vi "Autonomous Independent.vi"   [LabVIEW 2017]
doc: "This VI is called when autonomous begins, and will automatically be terminated when autonomous ends. You can carry out timed or sensor driven robot movement independently without needing to return to the caller."
uses:
  <vilib>/Rock Robotics/WPI/Utilities/WPI_GetSetVariantRefNum.vi
  <vilib>/Rock Robotics/Network Tables/NT Write Numeric Array.vi
  <vilib>/Rock Robotics/Network Tables/NT Read String.vi
  <vilib>/Rock Robotics/WPI/RobotDrive/WPI_RobotDriveMecanumDrive_Cartesian.vi
panel:
  # "Be sure to right-click and choose Data Operations>>Make Current Value default if you want to save the array values with the VI"
types:
  T1 = typedef "WPI_JoystickDevRef.ctl" = cluster{"Device":T2}
  T2 = typedef "WPI_JoystickDeviceEnum.ctl" = enum16{"USB 0", "USB 1", "USB 2", "USB 3", "USB 4", "USB 5"}
  T3 = typedef "WPI_RobotDriveDevRef.ctl" = cluster{"DevStatus":errorcluster, "Motors[]":T4[], "Square Inputs":bool, "Max Output":dbl}
  T4 = typedef "WPI_MotorControlDeviceRef.ctl" = cluster{"DeviceStatus":errorcluster, "Type":T5, "PWM":cluster{"PWM Channel":T6, "DeadBand":T7}, "CAN":cluster{"Device Number":u8, "SetOutput VI Ref":variant, "GetOutput VI Ref":variant, "Enable VI Ref":variant, "Disable VI Ref":variant, "Data":variant}, "Invert":bool, "DIO PWM":cluster{"PWM \"Enable\" Channel":T6, "DIOChannel":T8, "PWM Rate":dbl}}
  T5 = typedef "WPI_MotorControlType.ctl" = enum16{"PWM", "CAN", "DIO PWM"}
  T6 = typedef "FPGA_DIOPWMChannel.ctl" = enum8{"PWM 0", "PWM 1", "PWM 2", "PWM 3", "PWM 4", "PWM 5", "PWM 6", "PWM 7", "PWM 8", "PWM 9", "PWM MXP 0", "PWM MXP 1", "PWM MXP 2", "PWM MXP 3", "PWM MXP 4", "PWM MXP 5", "PWM MXP 6", "PWM MXP 7", "PWM MXP 8", "PWM MXP 9", "Invalid"}
  T7 = typedef "WPI_PWMDeadband.ctl" = cluster{"Name":string, "maxPositivePwm":i32, "minPositivePwm":i32, "centerPwm":i32, "maxNegativePwm":i32, "minNegativePwm":i32, "angularRange":u16}
  T8 = typedef "FPGA_DIOChannel.ctl" = enum8{"DIO 0", "DIO 1", "DIO 2", "DIO 3", "DIO 4", "DIO 5", "DIO 6", "DIO 7", "DIO 8", "DIO 9", "DIO MXP 0", "DIO MXP 1", "DIO MXP 2", "DIO MXP 3", "DIO MXP 4", "DIO MXP 5", "DIO MXP 6", "DIO MXP 7", "DIO MXP 8", "DIO MXP 9", "DIO MXP 10", "DIO MXP 11", "DIO MXP 12", "DIO MXP 13", "DIO MXP 14", "DIO MXP 15", "SPI Port CS1", "SPI Port CS2", "SPI Port CS3", "SPI Port MISO", "SPI Port MOSI", "Invalid"}
  T9 = cluster{"RobotDriveDevRef":T3, "error out":errorcluster}
  T10 = cluster{"RobotDriveDevRef 2":T3, "error out":errorcluster}
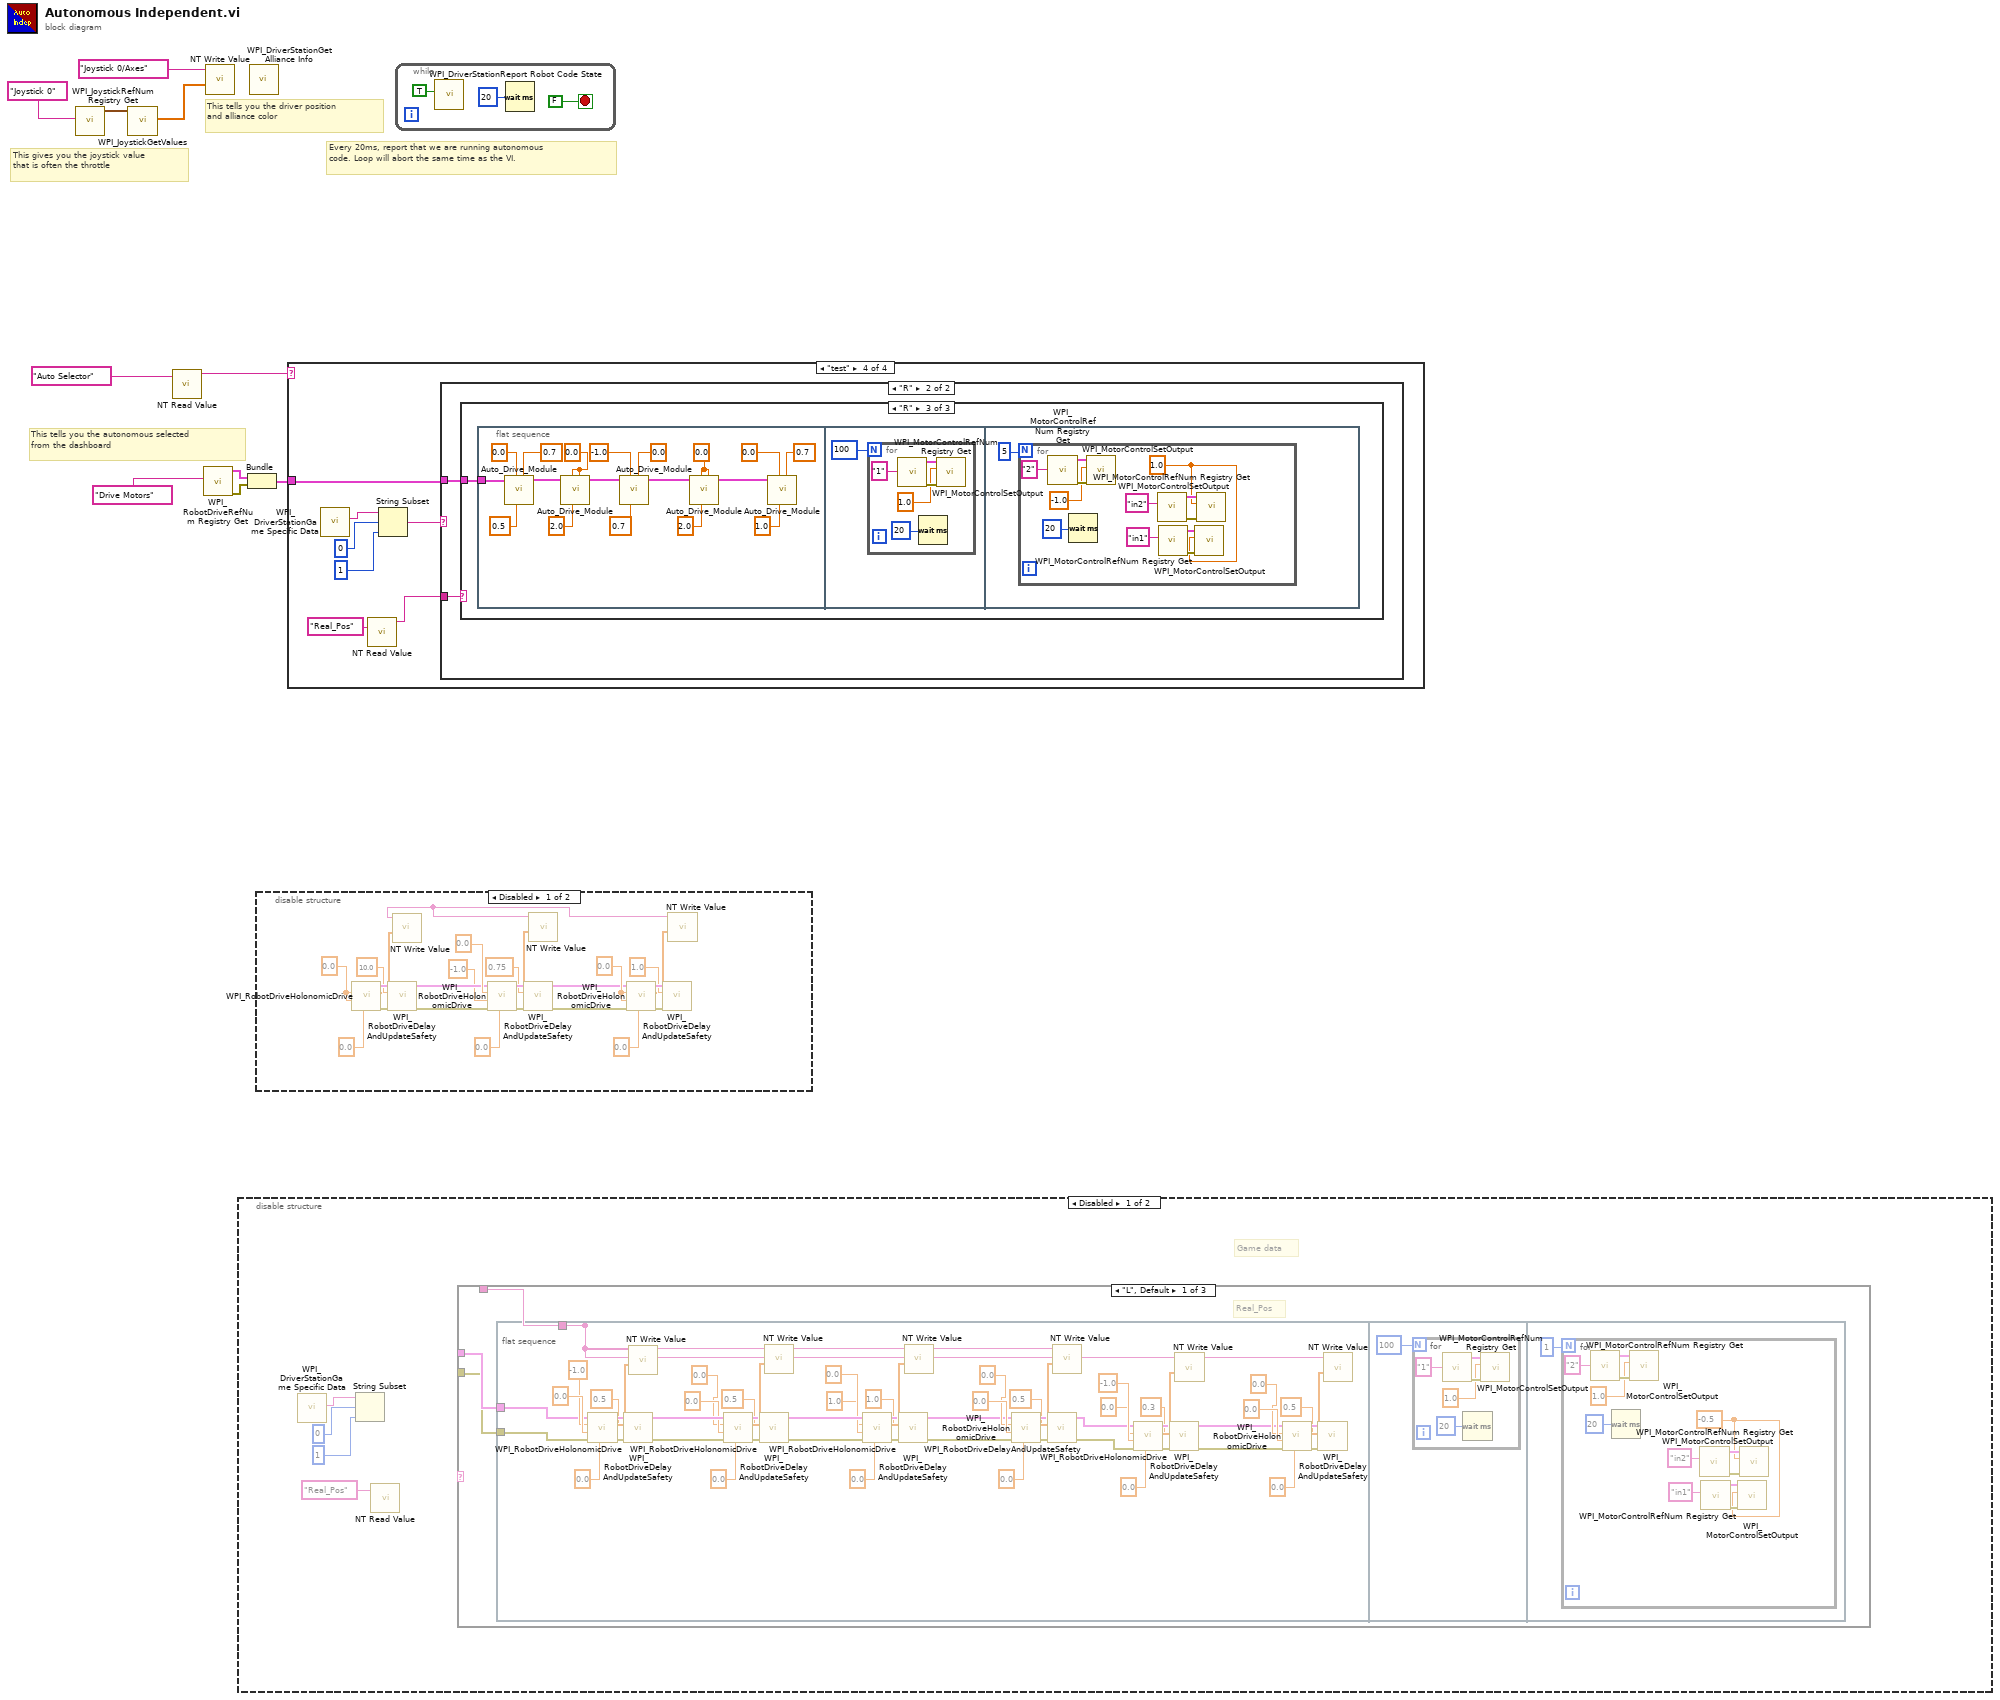
[diagram p0: block diagram]
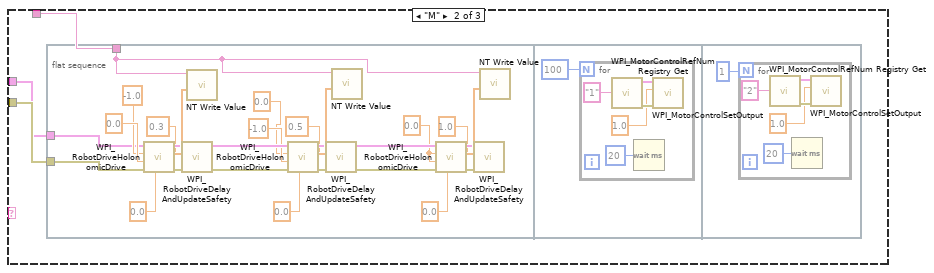
[diagram p2: hidden frame]
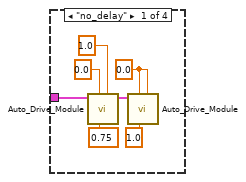
[diagram p6: hidden frame]
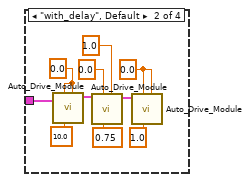
[diagram p7: hidden frame]
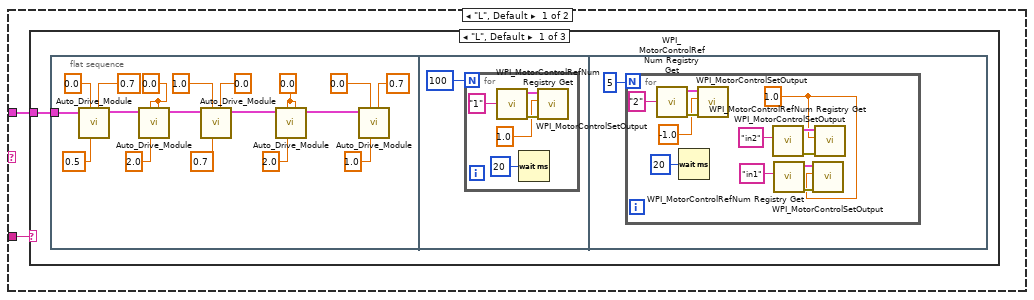
[diagram p9: hidden frame]
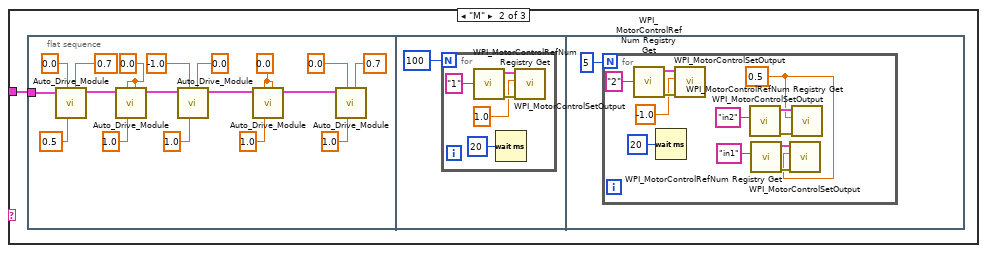
[diagram p10: hidden frame]
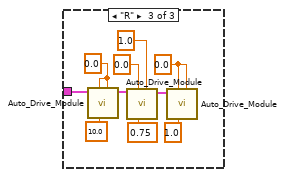
[diagram p11: hidden frame]
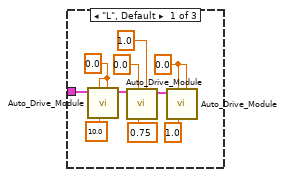
[diagram p12: hidden frame]
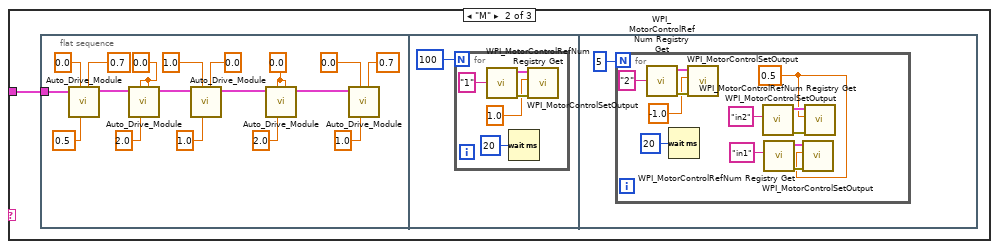
[diagram p13: hidden frame]
diagram:
  # "This tells you the autonomous selected\nfrom the dashboard"
  # "Every 20ms, report that we are running autonomous\ncode. Loop will abort the same time as the VI."
  # "This tells you the driver position\nand alliance color"
  # "This gives you the joystick value\nthat is often the throttle"
  n1 = call <vilib>:"WPI_JoystickRefNum Registry Get.vi"("refnum name"="Joystick 0") -> ("JoystickDevRef"=w8:T1)  [unwired: 1 in, 9 out]
  n2 = call <vilib>:"WPI_JoystickGetValues.vi"("JoystickDevRef"=w8) -> ("Axes"=w7:dbl[])  [unwired: 6 in, 4 out]
  n3 = call-poly <vilib>:"NT Read Value.vi"("Name"="Auto Selector") -> ("String"=w4:string)  [unwired: 9 in, 1 out]
  n4 = call <vilib>:"WPI_RobotDriveRefNum Registry Get.vi"("refnum name"="Drive Motors") -> ("error out"=w3:errorcluster, "RobotDriveDevRef"=w2:T3)  [unwired: 1 in, 8 out]
  n5 = call-poly <vilib>:"NT Write Value.vi"("Numeric Array"=w7, "Name"="Joystick 0/Axes") -> ()  [unwired: 9 in, 1 out]
  n6 = disable-structure shown="Disabled" {
    frame Disabled {
      # "Game data"
      n7 = call <vilib>:"WPI_DriverStationGame Specific Data.vi"() -> ("Game Specific Data"=w12:string)  [unwired: 11 in]
      n8 = String Subset(string=w12, offset (0)=0, length (rest)=1) -> ()  [unwired: 1 out]
      n9 = call-poly <vilib>:"NT Read Value.vi"("Name"="Real_Pos") -> ()  [unwired: 9 in, 2 out]
      n10 = case shown="\"L\", Default" {
        selector: _ -> [_ _ _]
        tunnel: _ -> [w15 w94 _]
        tunnel: _ -> [w16 w93 _]
        tunnel: _ -> [w17 w92 _]
        frame "L", Default {
          # "Real_Pos"
          n11 = flat-sequence {
            tunnel: w15 -> [w51]
            tunnel: w16 -> [w48]
            tunnel: [w19] -> _
            tunnel: w17 -> [w19]
            frame #0 {
              n12 = call-poly <vilib>:"WPI_RobotDriveHolonomicDrive.vi"("Rotation"=0.0, "error in (no error)"=w51, "Y"=0.0, "X"=-1.0, "RobotDriveDevRef"=w48) -> ("error out"=w60:errorcluster, "Motor Values"=w70:dbl[], "RobotDriveDevRef"=w61:T3)  [unwired: 4 in]
              n13 = call <vilib>:"WPI_RobotDriveDelayAndUpdateSafety.vi"("error in (no error)"=w60, "Delay (s)"=0.5, "RobotDriveDevRef"=w61) -> ("error out"=w65:errorcluster, "RobotDriveDevRef 2"=w64:T3)  [unwired: 7 in]
              n14 = call-poly <vilib>:"NT Write Value.vi"("Numeric Array"=w70, "Name"=w19) -> ()  [unwired: 9 in, 1 out]
              n15 = call-poly <vilib>:"WPI_RobotDriveHolonomicDrive.vi"("Rotation"=0.0, "error in (no error)"=w65, "Y"=0.0, "X"=0.0, "RobotDriveDevRef"=w64) -> ("error out"=w62:errorcluster, "Motor Values"=w71:dbl[], "RobotDriveDevRef"=w63:T3)  [unwired: 4 in]
              n16 = call <vilib>:"WPI_RobotDriveDelayAndUpdateSafety.vi"("error in (no error)"=w62, "Delay (s)"=0.5, "RobotDriveDevRef"=w63) -> ("error out"=w69:errorcluster, "RobotDriveDevRef 2"=w68:T3)  [unwired: 7 in]
              n17 = call-poly <vilib>:"NT Write Value.vi"("Numeric Array"=w71, "Name"=w19) -> ()  [unwired: 9 in, 1 out]
              n18 = call-poly <vilib>:"WPI_RobotDriveHolonomicDrive.vi"("Rotation"=0.0, "error in (no error)"=w69, "Y"=0.0, "X"=1.0, "RobotDriveDevRef"=w68) -> ("error out"=w66:errorcluster, "Motor Values"=w72:dbl[], "RobotDriveDevRef"=w67:T3)  [unwired: 4 in]
              n19 = call <vilib>:"WPI_RobotDriveDelayAndUpdateSafety.vi"("error in (no error)"=w66, "Delay (s)"=1.0, "RobotDriveDevRef"=w67) -> ("error out"=w39:errorcluster, "RobotDriveDevRef 2"=w40:T3)  [unwired: 7 in]
              n20 = call-poly <vilib>:"NT Write Value.vi"("Numeric Array"=w72, "Name"=w19) -> ()  [unwired: 9 in, 1 out]
              n21 = call-poly <vilib>:"WPI_RobotDriveHolonomicDrive.vi"("Rotation"=0.0, "error in (no error)"=w39, "Y"=0.0, "X"=0.0, "RobotDriveDevRef"=w40) -> ("error out"=w45:errorcluster, "Motor Values"=w47:dbl[], "RobotDriveDevRef"=w46:T3)  [unwired: 4 in]
              n22 = call <vilib>:"WPI_RobotDriveDelayAndUpdateSafety.vi"("error in (no error)"=w45, "Delay (s)"=0.5, "RobotDriveDevRef"=w46) -> ("error out"=w20:errorcluster, "RobotDriveDevRef 2"=w21:T3)  [unwired: 7 in]
              n23 = call-poly <vilib>:"NT Write Value.vi"("Numeric Array"=w47, "Name"=w19) -> ()  [unwired: 9 in, 1 out]
              n24 = call-poly <vilib>:"WPI_RobotDriveHolonomicDrive.vi"("Rotation"=0.0, "error in (no error)"=w20, "Y"=-1.0, "X"=0.0, "RobotDriveDevRef"=w21) -> ("error out"=w34:errorcluster, "Motor Values"=w36:dbl[], "RobotDriveDevRef"=w35:T3)  [unwired: 4 in]
              n25 = call <vilib>:"WPI_RobotDriveDelayAndUpdateSafety.vi"("error in (no error)"=w34, "Delay (s)"=0.3, "RobotDriveDevRef"=w35) -> ("error out"=w23:errorcluster, "RobotDriveDevRef 2"=w24:T3)  [unwired: 7 in]
              n26 = call-poly <vilib>:"NT Write Value.vi"("Numeric Array"=w36, "Name"=w19) -> ()  [unwired: 9 in, 1 out]
              n27 = call-poly <vilib>:"WPI_RobotDriveHolonomicDrive.vi"("Rotation"=0.0, "error in (no error)"=w23, "Y"=0.0, "X"=0.0, "RobotDriveDevRef"=w24) -> ("error out"=w29:errorcluster, "Motor Values"=w31:dbl[], "RobotDriveDevRef"=w30:T3)  [unwired: 4 in]
              n28 = call <vilib>:"WPI_RobotDriveDelayAndUpdateSafety.vi"("error in (no error)"=w29, "Delay (s)"=0.5, "RobotDriveDevRef"=w30) -> ()  [unwired: 7 in, 2 out]
              n29 = call-poly <vilib>:"NT Write Value.vi"("Numeric Array"=w31, "Name"=w19) -> ()  [unwired: 9 in, 1 out]
            }
            frame #1 {
              n30 = for {
                N: 100 -> [_]
                n31 = call <vilib>:"WPI_MotorControlRefNum Registry Get.vi"("refnum name"="1") -> ("error out"=w76:errorcluster, "MotorControlDevRef"=w75:T4)  [unwired: 9 in]
                n32 = Wait (ms)(milliseconds to wait=u32 20) -> ()  [unwired: 1 out]
                n33 = call <vilib>:"WPI_MotorControlSetOutput.vi"("error in (no error)"=w76, "Output"=1.0, "MotorControlDevRef"=w75) -> ()  [unwired: 6 in, 3 out]
              }
            }
            frame #2 {
              n34 = for {
                N: 1 -> [_]
                w82 = -0.5
                n35 = call <vilib>:"WPI_MotorControlRefNum Registry Get.vi"("refnum name"="2") -> ("error out"=w89:errorcluster, "MotorControlDevRef"=w87:T4)  [unwired: 9 in]
                n36 = Wait (ms)(milliseconds to wait=u32 20) -> ()  [unwired: 1 out]
                n37 = call <vilib>:"WPI_MotorControlSetOutput.vi"("error in (no error)"=w89, "Output"=1.0, "MotorControlDevRef"=w87) -> ()  [unwired: 6 in, 3 out]
                n38 = call <vilib>:"WPI_MotorControlRefNum Registry Get.vi"("refnum name"="in2") -> ("error out"=w84:errorcluster, "MotorControlDevRef"=w83:T4)  [unwired: 9 in]
                n39 = call <vilib>:"WPI_MotorControlRefNum Registry Get.vi"("refnum name"="in1") -> ("error out"=w86:errorcluster, "MotorControlDevRef"=w85:T4)  [unwired: 9 in]
                n40 = call <vilib>:"WPI_MotorControlSetOutput.vi"("error in (no error)"=w86, "Output"=w82, "MotorControlDevRef"=w85) -> ()  [unwired: 6 in, 3 out]
                n41 = call <vilib>:"WPI_MotorControlSetOutput.vi"("error in (no error)"=w84, "Output"=w82, "MotorControlDevRef"=w83) -> ()  [unwired: 6 in, 3 out]
              }
            }
          }
        }
        frame "M" {
          n42 = flat-sequence {
            tunnel: w94 -> [w99]
            tunnel: w93 -> [w96]
            tunnel: w92 -> [w95]
            frame #0 {
              w106 = 0.0
              n43 = call-poly <vilib>:"WPI_RobotDriveHolonomicDrive.vi"("Rotation"=0.0, "error in (no error)"=w99, "Y"=0.0, "X"=-1.0, "RobotDriveDevRef"=w96) -> ("error out"=w109:errorcluster, "Motor Values"=w119:dbl[], "RobotDriveDevRef"=w110:T3)  [unwired: 4 in]
              n44 = call <vilib>:"WPI_RobotDriveDelayAndUpdateSafety.vi"("error in (no error)"=w109, "Delay (s)"=0.3, "RobotDriveDevRef"=w110) -> ("error out"=w114:errorcluster, "RobotDriveDevRef 2"=w113:T3)  [unwired: 7 in]
              n45 = call-poly <vilib>:"NT Write Value.vi"("Numeric Array"=w119, "Name"=w95) -> ()  [unwired: 9 in, 1 out]
              n46 = call-poly <vilib>:"WPI_RobotDriveHolonomicDrive.vi"("Rotation"=0.0, "error in (no error)"=w114, "Y"=-1.0, "X"=0.0, "RobotDriveDevRef"=w113) -> ("error out"=w111:errorcluster, "Motor Values"=w120:dbl[], "RobotDriveDevRef"=w112:T3)  [unwired: 4 in]
              n47 = call <vilib>:"WPI_RobotDriveDelayAndUpdateSafety.vi"("error in (no error)"=w111, "Delay (s)"=0.5, "RobotDriveDevRef"=w112) -> ("error out"=w118:errorcluster, "RobotDriveDevRef 2"=w117:T3)  [unwired: 7 in]
              n48 = call-poly <vilib>:"NT Write Value.vi"("Numeric Array"=w120, "Name"=w95) -> ()  [unwired: 9 in, 1 out]
              n49 = call-poly <vilib>:"WPI_RobotDriveHolonomicDrive.vi"("Rotation"=0.0, "error in (no error)"=w118, "Y"=w106, "X"=w106, "RobotDriveDevRef"=w117) -> ("error out"=w115:errorcluster, "Motor Values"=w121:dbl[], "RobotDriveDevRef"=w116:T3)  [unwired: 4 in]
              n50 = call <vilib>:"WPI_RobotDriveDelayAndUpdateSafety.vi"("error in (no error)"=w115, "Delay (s)"=1.0, "RobotDriveDevRef"=w116) -> ()  [unwired: 7 in, 2 out]
              n51 = call-poly <vilib>:"NT Write Value.vi"("Numeric Array"=w121, "Name"=w95) -> ()  [unwired: 9 in, 1 out]
            }
            frame #1 {
              n52 = for {
                N: 100 -> [_]
                n53 = call <vilib>:"WPI_MotorControlRefNum Registry Get.vi"("refnum name"="1") -> ("error out"=w125:errorcluster, "MotorControlDevRef"=w124:T4)  [unwired: 9 in]
                n54 = Wait (ms)(milliseconds to wait=u32 20) -> ()  [unwired: 1 out]
                n55 = call <vilib>:"WPI_MotorControlSetOutput.vi"("error in (no error)"=w125, "Output"=1.0, "MotorControlDevRef"=w124) -> ()  [unwired: 6 in, 3 out]
              }
            }
            frame #2 {
              n56 = for {
                N: 1 -> [_]
                n57 = call <vilib>:"WPI_MotorControlRefNum Registry Get.vi"("refnum name"="2") -> ("error out"=w131:errorcluster, "MotorControlDevRef"=w129:T4)  [unwired: 9 in]
                n58 = Wait (ms)(milliseconds to wait=u32 20) -> ()  [unwired: 1 out]
                n59 = call <vilib>:"WPI_MotorControlSetOutput.vi"("error in (no error)"=w131, "Output"=1.0, "MotorControlDevRef"=w129) -> ()  [unwired: 6 in, 3 out]
              }
            }
          }
        }
        frame "R" {
        }
      }
    }
    frame Enabled {
    }
  }
  n60 = Bundle("RobotDriveDevRef"=w2, "error out"=w3) -> (w1:T9)  [unwired: 1 in]
  n61 = call <vilib>:"WPI_DriverStationGet Alliance Info.vi"() -> ()  [unwired: 12 out]
  n62 = disable-structure shown="Disabled" {
    frame Disabled {
      w140 = 0.0
      w153 = 0.0
      n63 = call-poly <vilib>:"WPI_RobotDriveHolonomicDrive.vi"("Rotation"=0.0, "Y"=w153, "X"=w153) -> ("error out"=w159:errorcluster, "Motor Values"=w137:dbl[], 3:"RobotDriveDevRef"=w158:T3, "error in (no error)"=w155:errorcluster, 11:"RobotDriveDevRef"=w154:T3)  [unwired: 4 in]
      n64 = call <vilib>:"WPI_RobotDriveDelayAndUpdateSafety.vi"("error in (no error)"=w159, "Delay (s)"=10.0, "RobotDriveDevRef"=w158) -> ("error out"=w146:errorcluster, "RobotDriveDevRef 2"=w147:T3)  [unwired: 7 in]
      n65 = call-poly <vilib>:"NT Write Value.vi"("Numeric Array"=w137) -> ("Name"=w134:string)  [unwired: 9 in, 1 out]
      n66 = call-poly <vilib>:"WPI_RobotDriveHolonomicDrive.vi"("Rotation"=0.0, "error in (no error)"=w146, "Y"=-1.0, "X"=0.0, "RobotDriveDevRef"=w147) -> ("error out"=w152:errorcluster, "Motor Values"=w136:dbl[], "RobotDriveDevRef"=w151:T3)  [unwired: 4 in]
      n67 = call <vilib>:"WPI_RobotDriveDelayAndUpdateSafety.vi"("error in (no error)"=w152, "Delay (s)"=0.75, "RobotDriveDevRef"=w151) -> ("error out"=w138:errorcluster, "RobotDriveDevRef 2"=w139:T3)  [unwired: 7 in]
      n68 = call-poly <vilib>:"NT Write Value.vi"("Numeric Array"=w136, "Name"=w134) -> ()  [unwired: 9 in, 1 out]
      n69 = call-poly <vilib>:"WPI_RobotDriveHolonomicDrive.vi"("Rotation"=0.0, "error in (no error)"=w138, "Y"=w140, "X"=w140, "RobotDriveDevRef"=w139) -> ("error out"=w144:errorcluster, "Motor Values"=w135:dbl[], "RobotDriveDevRef"=w143:T3)  [unwired: 4 in]
      n70 = call <vilib>:"WPI_RobotDriveDelayAndUpdateSafety.vi"("error in (no error)"=w144, "Delay (s)"=1.0, "RobotDriveDevRef"=w143) -> ()  [unwired: 7 in, 2 out]
      n71 = call-poly <vilib>:"NT Write Value.vi"("Numeric Array"=w135, "Name"=w134) -> ()  [unwired: 9 in, 1 out]
    }
    frame Enabled {
    }
  }
  n72 = case shown="\"test\"" w4 {
    tunnel: w1 -> [w160 w167 _ w177]
    frame "no_delay" {
      w161 = 0.0
      n73 = call "Auto_Drive_Module.vi"("Y"=1.0, "Lasting Time"=0.75, "X"=0.0, "DevRef & Err in"=w160) -> ("DevRef & Err out"=w166:T10)  [unwired: 7 in]
      n74 = call "Auto_Drive_Module.vi"("Y"=w161, "Lasting Time"=1.0, "X"=w161, "DevRef & Err in"=w166) -> ()  [unwired: 7 in, 1 out]
    }
    frame "with_delay", Default {
      w168 = 0.0
      w171 = 0.0
      n75 = call "Auto_Drive_Module.vi"("Y"=w171, "Lasting Time"=10.0, "X"=w171, "DevRef & Err in"=w167) -> ("DevRef & Err out"=w176:T10)  [unwired: 7 in]
      n76 = call "Auto_Drive_Module.vi"("Y"=1.0, "Lasting Time"=0.75, "X"=0.0, "DevRef & Err in"=w176) -> ("DevRef & Err out"=w175:T10)  [unwired: 7 in]
      n77 = call "Auto_Drive_Module.vi"("Y"=w168, "Lasting Time"=1.0, "X"=w168, "DevRef & Err in"=w175) -> ()  [unwired: 7 in, 1 out]
    }
    frame "stay" {
    }
    frame "test" {
      n78 = call <vilib>:"WPI_DriverStationGame Specific Data.vi"() -> ("Game Specific Data"=w181:string)  [unwired: 11 in]
      n79 = call-poly <vilib>:"NT Read Value.vi"("Name"="Real_Pos") -> ("String"=w178:string)  [unwired: 9 in, 1 out]
      n80 = String Subset(string=w181, offset (0)=0, length (rest)=1) -> (substring=w179:string)
      n81 = case shown="\"R\"" w179 {
        tunnel: w178 -> [w185 w273]
        tunnel: w177 -> [w184 w272]
        frame "L", Default {
          n82 = case shown="\"L\", Default" w185 {
            tunnel: w184 -> [w186 w224 w262]
            frame "L", Default {
              n83 = flat-sequence {
                tunnel: w186 -> [w204]
                frame #0 {
                  w189 = 0.0
                  w192 = 0.0
                  n84 = call "Auto_Drive_Module.vi"("Y"=0.7, "Lasting Time"=0.5, "X"=0.0, "DevRef & Err in"=w204) -> ("DevRef & Err out"=w194:T10)  [unwired: 7 in]
                  n85 = call "Auto_Drive_Module.vi"("Y"=w192, "Lasting Time"=2.0, "X"=w192, "DevRef & Err in"=w194) -> ("DevRef & Err out"=w193:T10)  [unwired: 7 in]
                  n86 = call "Auto_Drive_Module.vi"("Y"=0.0, "Lasting Time"=0.7, "X"=1.0, "DevRef & Err in"=w193) -> ("DevRef & Err out"=w187:T10)  [unwired: 7 in]
                  n87 = call "Auto_Drive_Module.vi"("Y"=w189, "Lasting Time"=2.0, "X"=w189, "DevRef & Err in"=w187) -> ("DevRef & Err out"=w188:T10)  [unwired: 7 in]
                  n88 = call "Auto_Drive_Module.vi"("Y"=0.7, "Lasting Time"=1.0, "X"=0.0, "DevRef & Err in"=w188) -> ()  [unwired: 7 in, 1 out]
                }
                frame #1 {
                  n89 = for {
                    N: 100 -> [_]
                    n90 = call <vilib>:"WPI_MotorControlRefNum Registry Get.vi"("refnum name"="1") -> ("error out"=w208:errorcluster, "MotorControlDevRef"=w207:T4)  [unwired: 9 in]
                    n91 = Wait (ms)(milliseconds to wait=u32 20) -> ()  [unwired: 1 out]
                    n92 = call <vilib>:"WPI_MotorControlSetOutput.vi"("error in (no error)"=w208, "Output"=1.0, "MotorControlDevRef"=w207) -> ()  [unwired: 6 in, 3 out]
                  }
                }
                frame #2 {
                  n93 = for {
                    N: 5 -> [_]
                    w214 = 1.0
                    n94 = call <vilib>:"WPI_MotorControlRefNum Registry Get.vi"("refnum name"="2") -> ("error out"=w221:errorcluster, "MotorControlDevRef"=w219:T4)  [unwired: 9 in]
                    n95 = Wait (ms)(milliseconds to wait=u32 20) -> ()  [unwired: 1 out]
                    n96 = call <vilib>:"WPI_MotorControlSetOutput.vi"("error in (no error)"=w221, "Output"=-1.0, "MotorControlDevRef"=w219) -> ()  [unwired: 6 in, 3 out]
                    n97 = call <vilib>:"WPI_MotorControlRefNum Registry Get.vi"("refnum name"="in2") -> ("error out"=w216:errorcluster, "MotorControlDevRef"=w215:T4)  [unwired: 9 in]
                    n98 = call <vilib>:"WPI_MotorControlRefNum Registry Get.vi"("refnum name"="in1") -> ("error out"=w218:errorcluster, "MotorControlDevRef"=w217:T4)  [unwired: 9 in]
                    n99 = call <vilib>:"WPI_MotorControlSetOutput.vi"("error in (no error)"=w218, "Output"=w214, "MotorControlDevRef"=w217) -> ()  [unwired: 6 in, 3 out]
                    n100 = call <vilib>:"WPI_MotorControlSetOutput.vi"("error in (no error)"=w216, "Output"=w214, "MotorControlDevRef"=w215) -> ()  [unwired: 6 in, 3 out]
                  }
                }
              }
            }
            frame "M" {
              n101 = flat-sequence {
                tunnel: w224 -> [w242]
                frame #0 {
                  w227 = 0.0
                  w230 = 0.0
                  n102 = call "Auto_Drive_Module.vi"("Y"=0.7, "Lasting Time"=0.5, "X"=0.0, "DevRef & Err in"=w242) -> ("DevRef & Err out"=w232:T10)  [unwired: 7 in]
                  n103 = call "Auto_Drive_Module.vi"("Y"=w230, "Lasting Time"=1.0, "X"=w230, "DevRef & Err in"=w232) -> ("DevRef & Err out"=w231:T10)  [unwired: 7 in]
                  n104 = call "Auto_Drive_Module.vi"("Y"=0.0, "Lasting Time"=1.0, "X"=-1.0, "DevRef & Err in"=w231) -> ("DevRef & Err out"=w225:T10)  [unwired: 7 in]
                  n105 = call "Auto_Drive_Module.vi"("Y"=w227, "Lasting Time"=1.0, "X"=w227, "DevRef & Err in"=w225) -> ("DevRef & Err out"=w226:T10)  [unwired: 7 in]
                  n106 = call "Auto_Drive_Module.vi"("Y"=0.7, "Lasting Time"=1.0, "X"=0.0, "DevRef & Err in"=w226) -> ()  [unwired: 7 in, 1 out]
                }
                frame #1 {
                  n107 = for {
                    N: 100 -> [_]
                    n108 = call <vilib>:"WPI_MotorControlRefNum Registry Get.vi"("refnum name"="1") -> ("error out"=w246:errorcluster, "MotorControlDevRef"=w245:T4)  [unwired: 9 in]
                    n109 = Wait (ms)(milliseconds to wait=u32 20) -> ()  [unwired: 1 out]
                    n110 = call <vilib>:"WPI_MotorControlSetOutput.vi"("error in (no error)"=w246, "Output"=1.0, "MotorControlDevRef"=w245) -> ()  [unwired: 6 in, 3 out]
                  }
                }
                frame #2 {
                  n111 = for {
                    N: 5 -> [_]
                    w252 = 0.5
                    n112 = call <vilib>:"WPI_MotorControlRefNum Registry Get.vi"("refnum name"="2") -> ("error out"=w259:errorcluster, "MotorControlDevRef"=w257:T4)  [unwired: 9 in]
                    n113 = Wait (ms)(milliseconds to wait=u32 20) -> ()  [unwired: 1 out]
                    n114 = call <vilib>:"WPI_MotorControlSetOutput.vi"("error in (no error)"=w259, "Output"=-1.0, "MotorControlDevRef"=w257) -> ()  [unwired: 6 in, 3 out]
                    n115 = call <vilib>:"WPI_MotorControlRefNum Registry Get.vi"("refnum name"="in2") -> ("error out"=w254:errorcluster, "MotorControlDevRef"=w253:T4)  [unwired: 9 in]
                    n116 = call <vilib>:"WPI_MotorControlRefNum Registry Get.vi"("refnum name"="in1") -> ("error out"=w256:errorcluster, "MotorControlDevRef"=w255:T4)  [unwired: 9 in]
                    n117 = call <vilib>:"WPI_MotorControlSetOutput.vi"("error in (no error)"=w256, "Output"=w252, "MotorControlDevRef"=w255) -> ()  [unwired: 6 in, 3 out]
                    n118 = call <vilib>:"WPI_MotorControlSetOutput.vi"("error in (no error)"=w254, "Output"=w252, "MotorControlDevRef"=w253) -> ()  [unwired: 6 in, 3 out]
                  }
                }
              }
            }
            frame "R" {
              w263 = 0.0
              w266 = 0.0
              n119 = call "Auto_Drive_Module.vi"("Y"=w266, "Lasting Time"=10.0, "X"=w266, "DevRef & Err in"=w262) -> ("DevRef & Err out"=w271:T10)  [unwired: 7 in]
              n120 = call "Auto_Drive_Module.vi"("Y"=1.0, "Lasting Time"=0.75, "X"=0.0, "DevRef & Err in"=w271) -> ("DevRef & Err out"=w270:T10)  [unwired: 7 in]
              n121 = call "Auto_Drive_Module.vi"("Y"=w263, "Lasting Time"=1.0, "X"=w263, "DevRef & Err in"=w270) -> ()  [unwired: 7 in, 1 out]
            }
          }
        }
        frame "R" {
          n122 = case shown="\"R\"" w273 {
            tunnel: w272 -> [w274 w284 w322]
            frame "L", Default {
              w275 = 0.0
              w278 = 0.0
              n123 = call "Auto_Drive_Module.vi"("Y"=w278, "Lasting Time"=10.0, "X"=w278, "DevRef & Err in"=w274) -> ("DevRef & Err out"=w283:T10)  [unwired: 7 in]
              n124 = call "Auto_Drive_Module.vi"("Y"=1.0, "Lasting Time"=0.75, "X"=0.0, "DevRef & Err in"=w283) -> ("DevRef & Err out"=w282:T10)  [unwired: 7 in]
              n125 = call "Auto_Drive_Module.vi"("Y"=w275, "Lasting Time"=1.0, "X"=w275, "DevRef & Err in"=w282) -> ()  [unwired: 7 in, 1 out]
            }
            frame "M" {
              n126 = flat-sequence {
                tunnel: w284 -> [w302]
                frame #0 {
                  w287 = 0.0
                  w290 = 0.0
                  n127 = call "Auto_Drive_Module.vi"("Y"=0.7, "Lasting Time"=0.5, "X"=0.0, "DevRef & Err in"=w302) -> ("DevRef & Err out"=w292:T10)  [unwired: 7 in]
                  n128 = call "Auto_Drive_Module.vi"("Y"=w290, "Lasting Time"=2.0, "X"=w290, "DevRef & Err in"=w292) -> ("DevRef & Err out"=w291:T10)  [unwired: 7 in]
                  n129 = call "Auto_Drive_Module.vi"("Y"=0.0, "Lasting Time"=1.0, "X"=1.0, "DevRef & Err in"=w291) -> ("DevRef & Err out"=w285:T10)  [unwired: 7 in]
                  n130 = call "Auto_Drive_Module.vi"("Y"=w287, "Lasting Time"=2.0, "X"=w287, "DevRef & Err in"=w285) -> ("DevRef & Err out"=w286:T10)  [unwired: 7 in]
                  n131 = call "Auto_Drive_Module.vi"("Y"=0.7, "Lasting Time"=1.0, "X"=0.0, "DevRef & Err in"=w286) -> ()  [unwired: 7 in, 1 out]
                }
                frame #1 {
                  n132 = for {
                    N: 100 -> [_]
                    n133 = call <vilib>:"WPI_MotorControlRefNum Registry Get.vi"("refnum name"="1") -> ("error out"=w306:errorcluster, "MotorControlDevRef"=w305:T4)  [unwired: 9 in]
                    n134 = Wait (ms)(milliseconds to wait=u32 20) -> ()  [unwired: 1 out]
                    n135 = call <vilib>:"WPI_MotorControlSetOutput.vi"("error in (no error)"=w306, "Output"=1.0, "MotorControlDevRef"=w305) -> ()  [unwired: 6 in, 3 out]
                  }
                }
                frame #2 {
                  n136 = for {
                    N: 5 -> [_]
                    w312 = 0.5
                    n137 = call <vilib>:"WPI_MotorControlRefNum Registry Get.vi"("refnum name"="2") -> ("error out"=w319:errorcluster, "MotorControlDevRef"=w317:T4)  [unwired: 9 in]
                    n138 = Wait (ms)(milliseconds to wait=u32 20) -> ()  [unwired: 1 out]
                    n139 = call <vilib>:"WPI_MotorControlSetOutput.vi"("error in (no error)"=w319, "Output"=-1.0, "MotorControlDevRef"=w317) -> ()  [unwired: 6 in, 3 out]
                    n140 = call <vilib>:"WPI_MotorControlRefNum Registry Get.vi"("refnum name"="in2") -> ("error out"=w314:errorcluster, "MotorControlDevRef"=w313:T4)  [unwired: 9 in]
                    n141 = call <vilib>:"WPI_MotorControlRefNum Registry Get.vi"("refnum name"="in1") -> ("error out"=w316:errorcluster, "MotorControlDevRef"=w315:T4)  [unwired: 9 in]
                    n142 = call <vilib>:"WPI_MotorControlSetOutput.vi"("error in (no error)"=w316, "Output"=w312, "MotorControlDevRef"=w315) -> ()  [unwired: 6 in, 3 out]
                    n143 = call <vilib>:"WPI_MotorControlSetOutput.vi"("error in (no error)"=w314, "Output"=w312, "MotorControlDevRef"=w313) -> ()  [unwired: 6 in, 3 out]
                  }
                }
              }
            }
            frame "R" {
              n144 = flat-sequence {
                tunnel: w322 -> [w340]
                frame #0 {
                  w325 = 0.0
                  w328 = 0.0
                  n145 = call "Auto_Drive_Module.vi"("Y"=0.7, "Lasting Time"=0.5, "X"=0.0, "DevRef & Err in"=w340) -> ("DevRef & Err out"=w330:T10)  [unwired: 7 in]
                  n146 = call "Auto_Drive_Module.vi"("Y"=w328, "Lasting Time"=2.0, "X"=w328, "DevRef & Err in"=w330) -> ("DevRef & Err out"=w329:T10)  [unwired: 7 in]
                  n147 = call "Auto_Drive_Module.vi"("Y"=0.0, "Lasting Time"=0.7, "X"=-1.0, "DevRef & Err in"=w329) -> ("DevRef & Err out"=w323:T10)  [unwired: 7 in]
                  n148 = call "Auto_Drive_Module.vi"("Y"=w325, "Lasting Time"=2.0, "X"=w325, "DevRef & Err in"=w323) -> ("DevRef & Err out"=w324:T10)  [unwired: 7 in]
                  n149 = call "Auto_Drive_Module.vi"("Y"=0.7, "Lasting Time"=1.0, "X"=0.0, "DevRef & Err in"=w324) -> ()  [unwired: 7 in, 1 out]
                }
                frame #1 {
                  n150 = for {
                    N: 100 -> [_]
                    n151 = call <vilib>:"WPI_MotorControlRefNum Registry Get.vi"("refnum name"="1") -> ("error out"=w344:errorcluster, "MotorControlDevRef"=w343:T4)  [unwired: 9 in]
                    n152 = Wait (ms)(milliseconds to wait=u32 20) -> ()  [unwired: 1 out]
                    n153 = call <vilib>:"WPI_MotorControlSetOutput.vi"("error in (no error)"=w344, "Output"=1.0, "MotorControlDevRef"=w343) -> ()  [unwired: 6 in, 3 out]
                  }
                }
                frame #2 {
                  n154 = for {
                    N: 5 -> [_]
                    w350 = 1.0
                    n155 = call <vilib>:"WPI_MotorControlRefNum Registry Get.vi"("refnum name"="2") -> ("error out"=w357:errorcluster, "MotorControlDevRef"=w355:T4)  [unwired: 9 in]
                    n156 = Wait (ms)(milliseconds to wait=u32 20) -> ()  [unwired: 1 out]
                    n157 = call <vilib>:"WPI_MotorControlSetOutput.vi"("error in (no error)"=w357, "Output"=-1.0, "MotorControlDevRef"=w355) -> ()  [unwired: 6 in, 3 out]
                    n158 = call <vilib>:"WPI_MotorControlRefNum Registry Get.vi"("refnum name"="in2") -> ("error out"=w352:errorcluster, "MotorControlDevRef"=w351:T4)  [unwired: 9 in]
                    n159 = call <vilib>:"WPI_MotorControlRefNum Registry Get.vi"("refnum name"="in1") -> ("error out"=w354:errorcluster, "MotorControlDevRef"=w353:T4)  [unwired: 9 in]
                    n160 = call <vilib>:"WPI_MotorControlSetOutput.vi"("error in (no error)"=w354, "Output"=w350, "MotorControlDevRef"=w353) -> ()  [unwired: 6 in, 3 out]
                    n161 = call <vilib>:"WPI_MotorControlSetOutput.vi"("error in (no error)"=w352, "Output"=w350, "MotorControlDevRef"=w351) -> ()  [unwired: 6 in, 3 out]
                  }
                }
              }
            }
          }
        }
      }
    }
  }
  n162 = while {
    stop <- FALSE stop-if-true
    n163 = call <vilib>:"WPI_DriverStationReport Robot Code State.vi"("Autonomous"=TRUE) -> ()  [unwired: 10 in, 1 out]
    n164 = Wait (ms)(milliseconds to wait=u32 20) -> ()  [unwired: 1 out]
  }
